vi "PmodTC1Read.vi"(7 "SPI Channel (0)":u8, 8 "error in (no error)":errorcluster, 10 "CS Channel":u8, 11 "LINX Resource in":T2) -> (0 "error out":errorcluster, 2 "Temperatures":T1, 3 "LINX Resource out":T2)   [LabVIEW 2014]
doc: "Read the specified SPI channel. SPI is full duplex, therefore the write and read operations take place simultaneously. \n\nThis VI outputs thermocouple and reference junction temperatures in Celsius.\n\nSPI Channel: specifies the device SPI channel to write/read to.\n\nCS Channel: the Chip Select (DIO) channel to use during the SPI transaction. The default CS channel is 10.\n\nCS Logic Level: specifies the logic level of the CS pin. Active low is most common and means that CS will idle high, then be driven low when a frame begins. All Data bytes are shifted out, then CS will be driven high to end the frame. PmodTC1 is active low."
uses:
  <vilib>/MakerHub/LINX/Private/Type Defs/LINX Ref.ctl
  <vilib>/MakerHub/LINX/Private/Type Defs/Platform.ctl
  <vilib>/MakerHub/LINX/Private/Type Defs/Interface.ctl
  <vilib>/MakerHub/LINX/Private/Device/Type Defs/LINX Device Config.ctl
  <vilib>/MakerHub/LINX/Private/Device/Type Defs/TCP Config.ctl
  <vilib>/MakerHub/LINX/Private/Device/Type Defs/Channels.ctl
  <vilib>/MakerHub/LINX/Public/Peripherals/SPI/SPI CS Config.ctl
  <vilib>/MakerHub/LINX/Private/Type Defs/Peripherals/SPI/SPI CS Logic Level.ctl
  <vilib>/MakerHub/LINX/Public/Peripherals/SPI/SPI Write Read 1 Frame.vi
  <vilib>/MakerHub/LINX/LMH-LINX.lvlib
  <vilib>/MakerHub/Toolbox/LMH-Toolbox.lvlib
  <vilib>/MakerHub/LINX/Private/Device/Device.lvlib
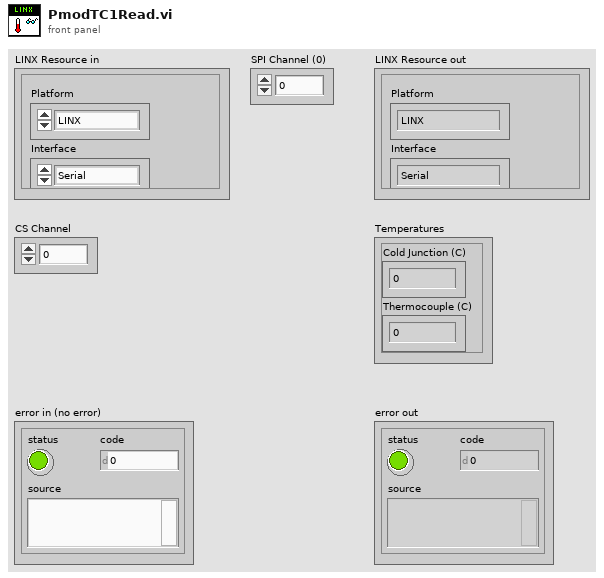
[diagram p1: front panel]
types:
  T1 = cluster{"Cold Junction (C)":i16, "Thermocouple (C)":i16}
  T2 = typedef "LMH-LINX.lvlib/LINX Ref.ctl" = cluster{"Platform":T3, "Interface":T4, "LINX Device Config":T5}
  T3 = typedef "LMH-LINX.lvlib/Platform.ctl" = enum16{"LINX", "myRIO"}
  T4 = typedef "LMH-LINX.lvlib/Interface.ctl" = enum16{"Serial", "TCP"}
  T5 = typedef "LMH-LINX.lvlib/Device.lvlib/LINX Device Config.ctl" = cluster{"Interface":T4, "COM Port":refnum<visa-resource-name>, "TCP Configuration":T6, "Device Family":u8, "Device ID":u8, "Device Name":string, "TCP Ref":refnum<k5>, "Channels":T7}
  T6 = typedef "LMH-LINX.lvlib/Device.lvlib/TCP Config.ctl" = cluster{"IP Address":string, "Port":u16}
  T7 = typedef "LMH-LINX.lvlib/Channels.ctl" = cluster{"DI":u8[], "DO":u8[], "AI":u8[], "AO":u8[], "PWM":u8[], "QE":u8[], "UART":u8[], "I2C 2":u8[], "SPI":u8[], "CAN":u8[], "Servo":u8[], "AI Ref (V)":dbl, "AO Ref (V)":dbl, "AO Resolution (Bits)":u8}
  T8 = typedef "LMH-LINX.lvlib/SPI CS Config.ctl" = cluster{"CS Channel":u8, "CS Logic Level":T9}
  T9 = typedef "LMH-LINX.lvlib/SPI CS Logic Level.ctl" = enum8{"Active Low", "Active High"}
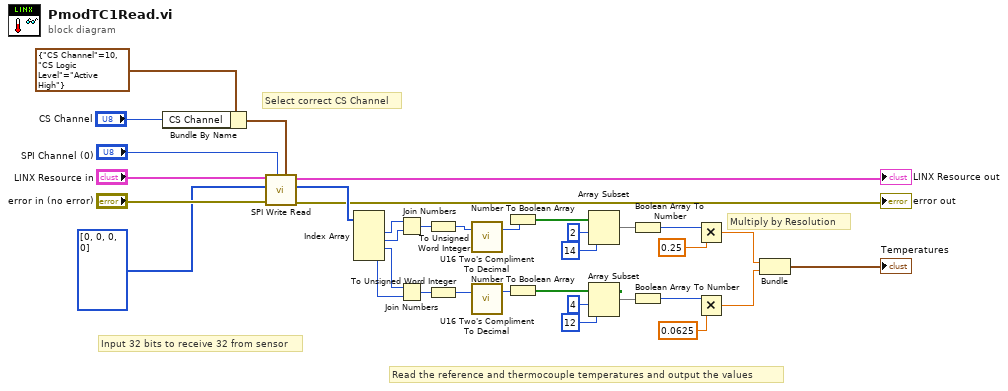
[diagram p0: block diagram]
diagram:
  # "Select correct CS Channel"
  # "Multiply by Resolution"
  # "Input 32 bits to receive 32 from sensor"
  # "Read the reference and thermocouple temperatures and output the values"
  n1 = Bundle By Name(cluster=T8 {"CS Channel"=10, "CS Logic Level"=enum."Active High"} ("CS Configuration"), "CS Channel"="CS Channel") -> (w25:T8)
  n2 = call-poly <vilib>:"SPI Write Read.vi"("CS Configuration"=w25, "SPI Channel (0)"="SPI Channel (0)", "Error In"="error in (no error)", "Data"=u8[] [0, 0, 0, 0], "LINX Resource"="LINX Resource in") -> ("Error Out"=→"error out":errorcluster, "Read Data"=w31:u8[], "LINX Resource"=→"LINX Resource out":T2)  [unwired: 4 in]
  n3 = Index Array(array=w31) -> (element #1=w13:u8, element #2=w12:u8, element #3=w10:u8, element #4=w9:u8)  [unwired: 4 in]
  n4 = Join Numbers(hi=w13, lo=w12) -> ((hi.lo)=w30:u16)
  n5 = Join Numbers(hi=w10, lo=w9) -> ((hi.lo)=w32:u16)
  n6 = To Unsigned Word Integer(number=w30) -> (unsigned 16bit integer=w16:u16)
  n7 = To Unsigned Word Integer(number=w32) -> (unsigned 16bit integer=w7:u16)
  n8 = call <vilib>:"U16 Two's Compliment To Decimal.vi"("Two's Compliment U16"=w16) -> ("Decimal I16"=w15:i16)  [unwired: 2 in]
  n9 = call <vilib>:"U16 Two's Compliment To Decimal.vi"("Two's Compliment U16"=w7) -> ("Decimal I16"=w4:i16)  [unwired: 2 in]
  n10 = Number To Boolean Array(number=w15) -> (Boolean array=w18:bool[])
  n11 = Number To Boolean Array(number=w4) -> (Boolean array=w2:bool[])
  n12 = Array Subset(array=w18, index=2, length=14) -> (w17:bool[])
  n13 = Array Subset(array=w2, index=4, length=12) -> (w1:bool[])
  n14 = Boolean Array To Number(Boolean array=w17) -> (number=w14:i16)
  n15 = Boolean Array To Number(Boolean array=w1) -> (number=w3:i16)
  n16 = Multiply(x=w14, y=0.25) -> (x*y=w22:dbl)
  n17 = Multiply(x=w3, y=0.0625) -> (x*y=w23:dbl)
  n18 = Bundle(w22, w23) -> (→"Temperatures":cluster{dbl, dbl})  [unwired: 1 in]
